vi "Save Macro Steps.vi"(8 "error in (no error)":errorcluster, 10 "Macro Steps":T1[](array[typedef]), 11 "refnum":T3) -> (0 "error out":errorcluster, 3 "refnum out":T3)   [LabVIEW 2023]
doc: "Saves the list of steps to the macro config file defined by <B>refnum</B>."
uses:
  <vilib>/Utility/config.llb/Config Data RefNum.ctl
  CTLs/Step V3.ctl
  CTLs/Step Type V3.ctl
  <vilib>/Utility/config.llb/Write Key (I32).vi
  <vilib>/Utility/config.llb/Write Key (String).vi
  <vilib>/Utility/config.llb/Write Key (Boolean).vi
  <vilib>/Utility/config.llb/Write Key (U32).vi
  <vilib>/Utility/config.llb/NI_LVConfig.lvlib
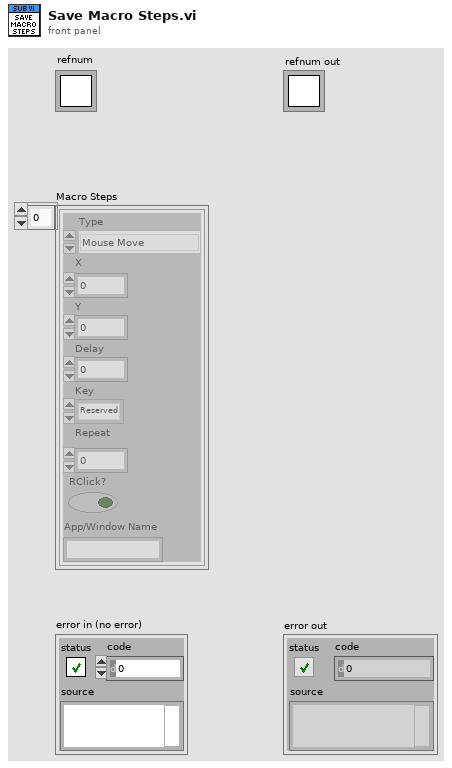
[diagram p1: front panel]
types:
  T1 = typedef "Step V3.ctl" = cluster{"Type":T2, "X":i32, "Y":i32, "Delay":i32, "Key":u8, "Repeat":i32, "RClick?":bool, "App/Window Name":string}
  T2 = typedef "Step Type V3.ctl" = enum16{"Mouse Move", "Mouse Click", "Key Press", "Wait", "Mouse Down", "Mouse Up", "Key Down", "Key Up", "Run Application", "Maximize Window", "Minimize Window", "Close Window", "Bring Window to Front", "Send Window to Back"}
  T3 = typedef "NI_LVConfig.lvlib/Config Data RefNum.ctl" = refnum<k1>
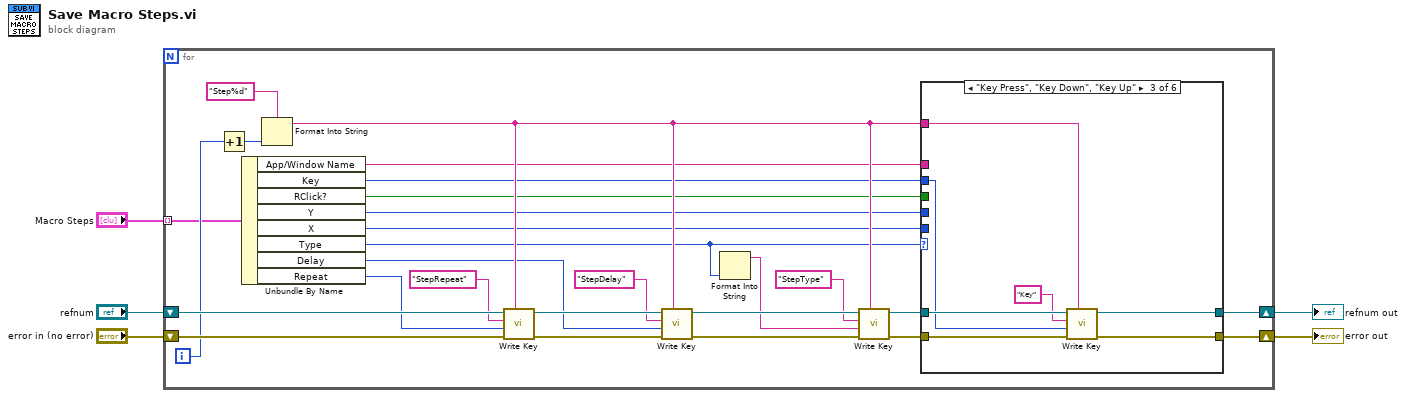
[diagram p0: block diagram]
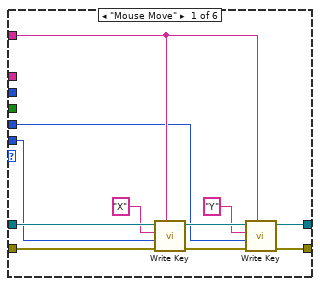
[diagram p2: hidden frame]
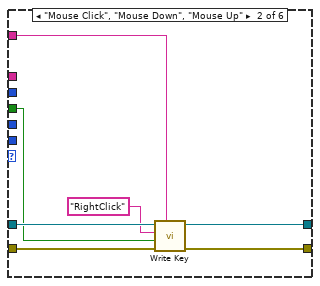
[diagram p3: hidden frame]
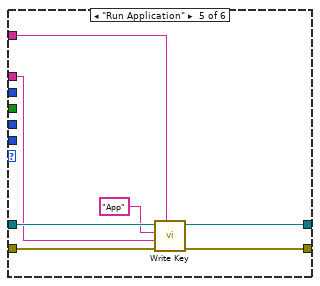
[diagram p5: hidden frame]
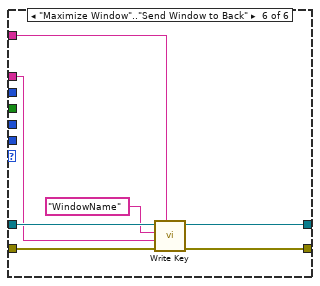
[diagram p6: hidden frame]
diagram:
  n1 = for {
    shift-right: [w24] -> w2
    shift-left: "error in (no error)" -> [w30]
    shift-right: [w23] -> w1
    shift-left: "refnum" -> [w27]
    tunnel: "Macro Steps" -> [w11] mode=indexing
    i -> [w21]
    n2 = Increment(x=w21) -> (x+1=w20:i32)
    n3 = Unbundle By Name(w11) -> ("App/Window Name"=w6:string, "Key"=w7:u8, "RClick?"=w8:bool, "Y"=w9:i32, "X"=w10:i32, "Type"=w16:T2, "Delay"=w12:i32, "Repeat"=w13:i32)
    n4 = Format Into String(format string="Step%d", w20) -> (resulting string=w32:string)  [unwired: 2 in, 1 out]
    n5 = call-poly <vilib>:"Write Key.vi"("section"=w32, "error in (no error)"=w30, "value"=w13, "key"="StepRepeat", "refnum"=w27) -> ("error out"=w31:errorcluster, "refnum out"=w28:T3)  [unwired: 4 in, 1 out]
    n6 = call-poly <vilib>:"Write Key.vi"("section"=w32, "error in (no error)"=w31, "value"=w12, "key"="StepDelay", "refnum"=w28) -> ("error out"=w29:errorcluster, "refnum out"=w26:T3)  [unwired: 4 in, 1 out]
    n7 = Format Into String(w16) -> (resulting string=w18:string)  [unwired: 3 in, 1 out]
    n8 = call-poly <vilib>:"Write Key.vi"("section"=w32, "error in (no error)"=w29, "value"=w18, "key"="StepType", "refnum"=w26) -> ("error out"=w15:errorcluster, "refnum out"=w14:T3)  [unwired: 4 in, 1 out]
    n9 = case shown="\"Key Press\", \"Key Down\", \"Key Up\"" w16 {
      tunnel: w15 -> [w42 w50 w57 w58 w66 w73]
      tunnel: w14 -> [w41 w49 w56 w59 w65 w72]
      tunnel: w32 -> [w37 w47 w54 _ w63 w70]
      tunnel: [w36 w45 w52 w58 w61 w68] -> w24
      tunnel: [w35 w46 w53 w59 w62 w69] -> w23
      tunnel: w10 -> [w34 _ _ _ _ _]
      tunnel: w9 -> [w33 _ _ _ _ _]
      tunnel: w8 -> [_ w44 _ _ _ _]
      tunnel: w7 -> [_ _ w51 _ _ _]
      tunnel: w6 -> [_ _ _ _ w60 w67]
      frame "Mouse Move" {
        n10 = call-poly <vilib>:"Write Key.vi"("section"=w37, "error in (no error)"=w42, "value"=w34, "key"="X", "refnum"=w41) -> ("error out"=w38:errorcluster, "refnum out"=w43:T3)  [unwired: 4 in, 1 out]
        n11 = call-poly <vilib>:"Write Key.vi"("section"=w37, "error in (no error)"=w38, "value"=w33, "key"="Y", "refnum"=w43) -> ("error out"=w36:errorcluster, "refnum out"=w35:T3)  [unwired: 4 in, 1 out]
      }
      frame "Mouse Click", "Mouse Down", "Mouse Up" {
        n12 = call-poly <vilib>:"Write Key.vi"("section"=w47, "error in (no error)"=w50, "value"=w44, "key"="RightClick", "refnum"=w49) -> ("error out"=w45:errorcluster, "refnum out"=w46:T3)  [unwired: 4 in, 1 out]
      }
      frame "Key Press", "Key Down", "Key Up" {
        n13 = call-poly <vilib>:"Write Key.vi"("section"=w54, "error in (no error)"=w57, "value"=w51, "key"="Key", "refnum"=w56) -> ("error out"=w52:errorcluster, "refnum out"=w53:T3)  [unwired: 4 in, 1 out]
      }
      frame "Wait" {
      }
      frame "Run Application" {
        n14 = call-poly <vilib>:"Write Key.vi"("section"=w63, "error in (no error)"=w66, "value"=w60, "key"="App", "refnum"=w65) -> ("error out"=w61:errorcluster, "refnum out"=w62:T3)  [unwired: 4 in, 1 out]
      }
      frame "Maximize Window".."Send Window to Back" {
        n15 = call-poly <vilib>:"Write Key.vi"("section"=w70, "error in (no error)"=w73, "value"=w67, "key"="WindowName", "refnum"=w72) -> ("error out"=w68:errorcluster, "refnum out"=w69:T3)  [unwired: 4 in, 1 out]
      }
    }
  }
  "error out" <- w2
  "refnum out" <- w1
